vi "GetCurrentCellData.vi"(8 "error in (no error)":errorcluster, 10 "ColumnIndex":i32, 11 "AdjustableMulticolumnListbox in":refnum<class "AdjMCLB.lvclass">) -> (0 "error out":errorcluster, 2 "Data":string, 3 "AdjustableMulticolumnListbox out":refnum<class "AdjMCLB.lvclass">)   [LabVIEW 2020, in "AdjMCLB.lvclass"]
uses:
  AdjMCLB.lvclass
  <vilib>/Utility/Data Type/NI_Data Type.lvlib
  <vilib>/ErrorRing/Error Ring.xnode
  <vilib>/Utility/error.llb/Error Cluster From Error Code.vi
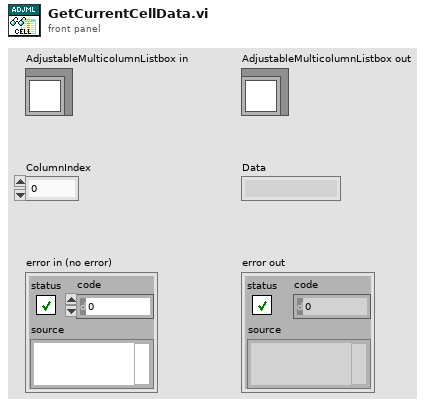
[diagram p1: front panel]
types:
  T1 = typedef "NI_Data Type.lvlib/Data Type.ctl" = enum8{"Invalid Type", "Void", "I8", "I16", "I32", "I64", "U8", "U16", "U32", "U64", "Single Float", "Double Float", "Extended Float", "Single Complex", "Double Complex", "Extended Complex", "Enum U8", "Enum U16", "Enum U32", "Enum U64", "Single Float With Unit", "Double Float With Unit", "Extended Float With Unit", "Single Complex with Unit", "Double Complex with Unit", "Extended Complex with Unit", "Boolean", "String", "Path", "Picture", "Tag", "Array", "Cluster", "Variant", "LV Variant", "Waveform", "Timestamp", "Digital Waveform", "Digital Data", "ExpressData", "Refnum", "External Data", "VI", "Poly VI", "LabVIEW Class Instance", "Fixed Point", "Set Collection", "Map Collection"}
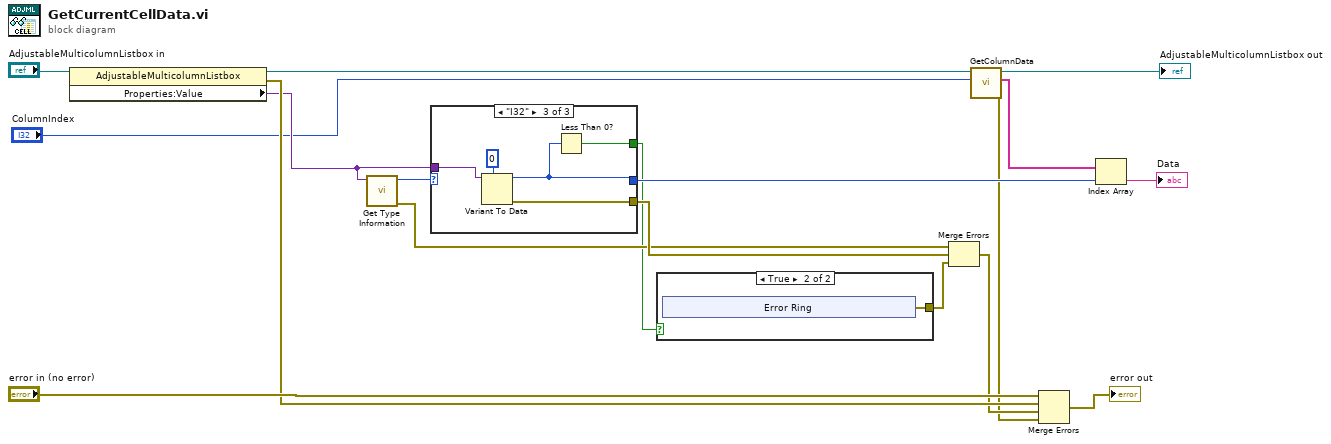
[diagram p0: block diagram]
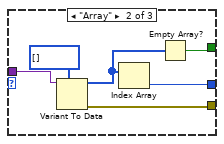
[diagram p4: hidden frame]
diagram:
  n1 = property class="AdjustableMulticolumnListbox"(reference="AdjustableMulticolumnListbox in") -> (reference out=w6:refnum<class "AdjMCLB.lvclass">, error out=w15:errorcluster, "Properties:Value"=w12:variant)  [unwired: 1 in]
  n2 = call <vilib>:"Get Type Information.vi"("variant"=w12) -> ("error out"=w10:errorcluster, "type"=w13:T1)  [unwired: 6 in, 3 out]
  n3 = case shown="\"I32\"" w13 {
    tunnel: w12 -> [_ w19 w28]
    tunnel: [_ w23 w27] -> w11
    tunnel: [_ w22 w26] -> w9
    tunnel: [_ w21 w25] -> w3
    frame Default {
    }
    frame "Array" {
      n4 = Variant To Data(type=i32[] [], Variant=w19) -> (data=w20:i32[], error out=w23:errorcluster)  [unwired: 1 in]
      n5 = Index Array(array=w20) -> (element=w22:i32)  [unwired: 1 in]
      n6 = Empty Array?(array=w20) -> (empty?=w21:bool)
    }
    frame "I32" {
      n7 = Variant To Data(type=0, Variant=w28) -> (data=w26:i32, error out=w27:errorcluster)  [unwired: 1 in]
      n8 = Less Than 0?(x=w26) -> (x < 0?=w25:bool)
    }
  }
  n9 = case shown="True" w3 {
    tunnel: [_ w30] -> w2
    frame False {
    }
    frame True {
      n10 = xnode "Error Ring"() -> ("error out"=w30:errorcluster)
    }
  }
  n11 = Merge Errors(w10, w11, w2) -> (w8:errorcluster)
  n12 = call-dynamic "GetColumnData.vi"("Index"="ColumnIndex", "AdjustableMulticolumnListbox in"=w6) -> ("error out"=w1:errorcluster, "ColumnData"=w4:string[], "AdjustableMulticolumnListbox out"=→"AdjustableMulticolumnListbox out":refnum<class "AdjMCLB.lvclass">)  [unwired: 7 in]
  n13 = Merge Errors("error in (no error)", w15, w8, w1) -> (→"error out":errorcluster)
  n14 = Index Array(array=w4, index=w9) -> (element=→"Data":string)
